vi "DSF.Engine.Transfer.Set Channel Blocks.vi"(10 "channel blocks":T1[](array[typedef]) {"buffer offset" format="%d bytes"}, 11 "Transfer in":refnum<class "DSF.Engine.Transfer.lvclass">) -> (3 "Transfer out":refnum<class "DSF.Engine.Transfer.lvclass">)   [LabVIEW 2017, in "Data Sharing Framework Engine.lvlib" / "DSF.Engine.Transfer.lvclass"]
uses:
  DSF.Engine.Transfer.lvclass
  Source/Data Sharing Framework Core/Engine/Type Definitions/DSF Runtime Channel Block.ctl
  Source/Data Sharing Framework Core/Configuration/1.0.0/Public/Controls/DSF Data Type.ctl
  DSF.Engine.Transfer.lvclass/DSF.Engine.Transfer.ctl
  Source/Data Sharing Framework Core/Engine/Data Sharing Framework Engine.lvlib
  Source/Data Sharing Framework Core/Configuration/1.0.0/Data Sharing Framework Configuration.lvlib
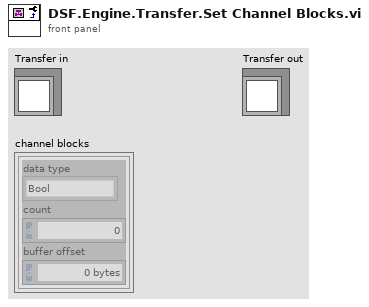
[diagram p1: front panel]
types:
  T1 = typedef "Data Sharing Framework Engine.lvlib/DSF Runtime Channel Block.ctl" = cluster{"data type":T2, "count":u64, "buffer offset":u64}
  T2 = typedef "Data Sharing Framework Configuration.lvlib/DSF Data Type.ctl" = enum8{"Bool", "SGL", "DBL", "I8", "I16", "I32", "I64", "U8", "U16", "U32", "U64"}
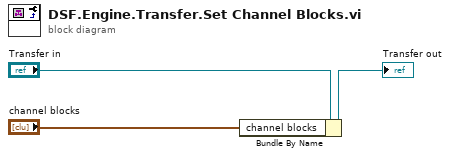
[diagram p0: block diagram]
diagram:
  n1 = Bundle By Name(cluster="Transfer in", "channel blocks"="channel blocks") -> (→"Transfer out":refnum<class "DSF.Engine.Transfer.lvclass">)
